vi "TcpDataProcessing.vi"(8 "TestPCアドレス":string) -> (4 "TestData":T2, 6 "Read Log":T3(array[cluster]))   [LabVIEW 2021]
uses:
  HallMeasurementStatus.ctl
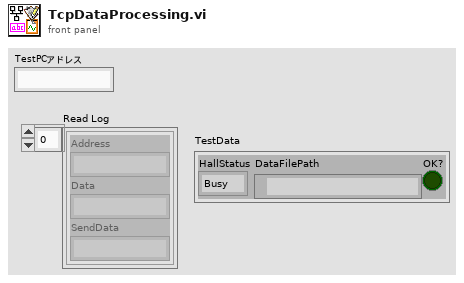
[diagram p1: front panel]
types:
  T1 = typedef "HallMeasurementStatus.ctl" = enum16{"Busy", "Ready", "Done", "Error"}
  T2 = cluster{"HallStatus":T1, "DataFilePath":path, "OK?":bool}
  T3 = cluster{"Address":string, "Data":string, "SendData":string}[]
  T4 = cluster{"アドレス":string, "Data":string, "SendData":string}[]
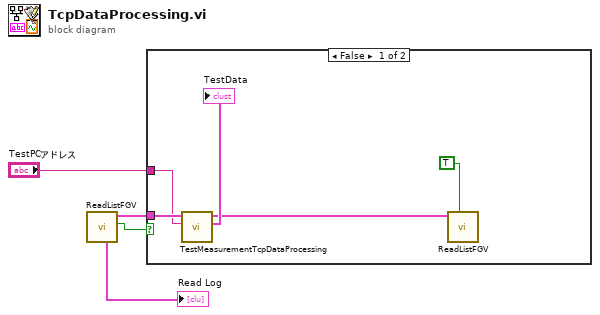
[diagram p0: block diagram]
diagram:
  n1 = call "ReadListFGV.vi"() -> ("空?"=w4:bool, "Read List Out"=w3:T3, "Read Log"=→"Read Log":T4)  [unwired: 9 in]
  n2 = case shown="False" w4 {
    tunnel: w3 -> [w8 _]
    tunnel: "TestPCアドレス" -> [w7 _]
    frame False {
      n3 = call "TestMeasurementTcpDataProcessing.vi"("Address"=w7, "Read Data"=w8) -> ("Data"=→"TestData":T2, "Read Data Out"=w5:T3)  [unwired: 8 in]
      n4 = call "ReadListFGV.vi"("Set"=TRUE, "Read Data"=w5) -> ()  [unwired: 7 in, 3 out]
    }
    frame True {
    }
  }
